vi "AppendStacks.vi"(10 "Second":refnum<class "Stack.lvclass">, 11 "First":refnum<class "Stack.lvclass">) -> (3 "First":refnum<class "Stack.lvclass">)   [LabVIEW 2024, in "ActionStack.lvlib" / "Stack.lvclass"]
uses:
  Stack.lvclass
  Stack.lvclass/Stack.ctl
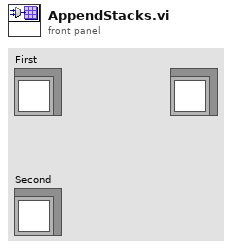
[diagram p1: front panel]
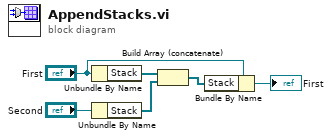
[diagram p0: block diagram]
diagram:
  n1 = Unbundle By Name("First") -> ("Stack"=w3:refnum<class "Action.lvclass">[])
  n2 = Unbundle By Name("Second") -> ("Stack"=w1:refnum<class "Action.lvclass">[])
  n3 = Build Array (concatenate)(w3, w1) -> (w2:refnum<class "Action.lvclass">[])
  n4 = Bundle By Name(cluster="First", "Stack"=w2) -> (→"First":refnum<class "Stack.lvclass">)
